vi "Release_Main.vi"(8 "Error in":errorcluster, 11 "Queues":T1) -> ()   [LabVIEW 2021, in "Queues.lvlib"]
doc: "This VI is used to destroy the queues, notifiers, user events of the Main VI."
uses:
  Queues.lvlib
  Tipski Definicii/Kalibrator_Sostojbi.ctl
  Tipski Definicii/QMH_Daq_States.ctl
panel:
  # "Input"
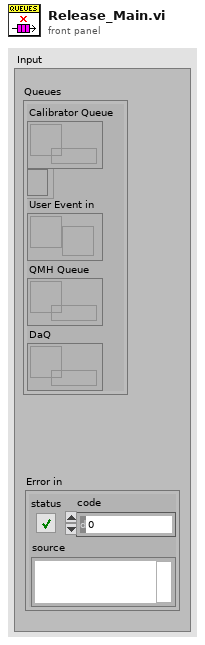
[diagram p1: front panel]
types:
  T1 = cluster{"Calibrator Queue ":refnum<queue>, "ER Refnum":refnum<event-registration>, "User Event in":refnum<user-event>, "QMH Queue ":refnum<queue>, "DaQ":refnum<queue>}
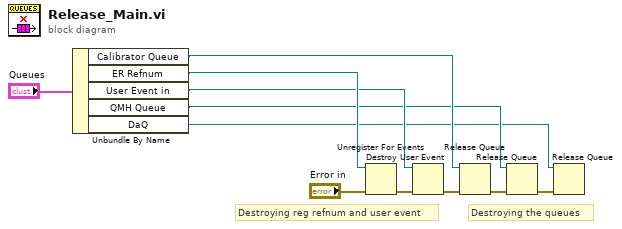
[diagram p0: block diagram]
diagram:
  # "Destroying the queues"
  # "Destroying reg refnum and user event"
  n1 = Unbundle By Name("Queues") -> ("Calibrator Queue"=w5:refnum<queue>, "ER Refnum"=w4:refnum<event-registration>, "User Event in"=w3:refnum<user-event>, "QMH Queue"=w2:refnum<queue>, "DaQ"=w1:refnum<queue>)
  n2 = Unregister For Events(event registration refnum=w4, error in="Error in") -> (error out=w7:errorcluster)
  n3 = Destroy User Event(user event=w3, error in=w7) -> (error out=w8:errorcluster)
  n4 = Release Queue(queue=w5, error in (no error)=w8) -> (error out=w9:errorcluster)  [unwired: 1 in, 2 out]
  n5 = Release Queue(queue=w2, error in (no error)=w9) -> (error out=w11:errorcluster)  [unwired: 1 in, 2 out]
  n6 = Release Queue(queue=w1, error in (no error)=w11) -> ()  [unwired: 1 in, 3 out]
